vi "Read Path.vi"(11 "ConfigManager.Text in":refnum<class "ConfigManager.Text.lvclass">) -> (2 "Path":path, 3 "ConfigManager.Text out":refnum<class "ConfigManager.Text.lvclass">)   [LabVIEW 2013, in "CfgManager.Text.lvlib" / "ConfigManager.Text.lvclass"]
uses:
  ConfigManager.Text.lvclass
  Manager/ConfigManager.lvclass/ConfigManager.ctl
  Manager/ConfigManager.lvclass
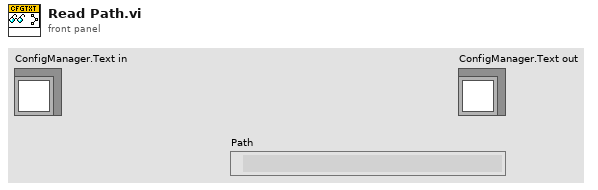
[diagram p1: front panel]
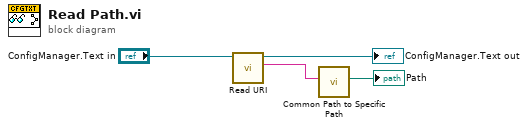
[diagram p0: block diagram]
diagram:
  n1 = call "Read URI.vi"("ConfigManager in"="ConfigManager.Text in") -> ("URI"=w2:string, "ConfigManager out"=→"ConfigManager.Text out":refnum<class "ConfigManager.Text.lvclass">)  [unwired: 9 in]
  n2 = call "Common Path to Specific Path.vi"("common path"=w2) -> ("specific path"=→"Path":path)  [unwired: 10 in]
